vi "VI Tree.vi"   [LabVIEW 2010, in "Fluke 884X Series.lvlib"]
doc: "This is the instrument driver for the Fluke 8845 and 8846 digital multimeter."
uses:
  <instrlib>/Fluke 884X Series/Fluke 884X Series.lvlib
  <instrlib>/Fluke 884X Series/Public/Data/Read (Multiple Points).vi
panel:
  # "(c) 2007 National Instruments.  ALL RIGHTS RESERVED."
  # "SEE DIAGRAM\nFOR VI Tree"
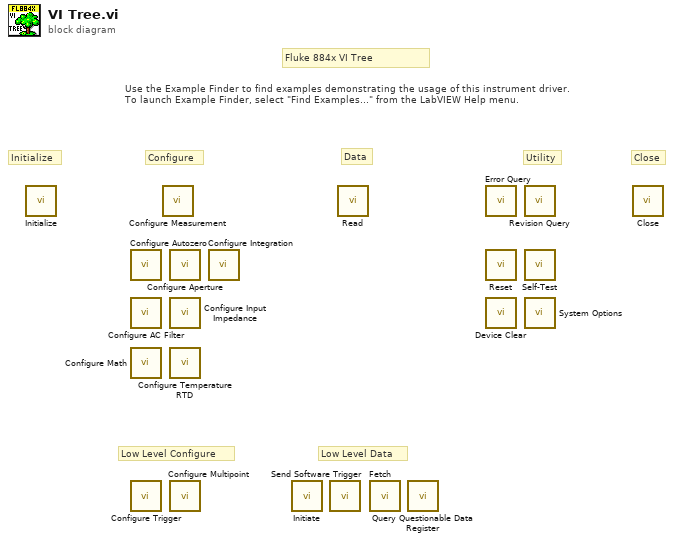
[diagram p0: block diagram]
diagram:
  # "Use the Example Finder to find examples demonstrating the usage of this instrument driver.\nTo launch Example Finder, select \"Find Examples...\" from the LabVIEW Help menu."
  # "Fluke 884x VI Tree"
  # "Low Level Configure"
  # "Low Level Data"
  # "Configure"
  # "Utility"
  # "Data"
  # "Close"
  # "Initialize"
  n1 = call <instrlib>:"Initialize.vi"() -> ()  [unwired: 10 in, 2 out]
  n2 = call <instrlib>:"Configure Autozero.vi"() -> ()  [unwired: 10 in, 2 out]
  n3 = call <instrlib>:"Configure AC Filter.vi"() -> ()  [unwired: 10 in, 2 out]
  n4 = call <instrlib>:"Configure Math.vi"() -> ()  [unwired: 14 in, 2 out]
  n5 = call <instrlib>:"Configure Trigger.vi"() -> ()  [unwired: 10 in, 2 out]
  n6 = call <instrlib>:"Configure Measurement.vi"() -> ()  [unwired: 10 in, 2 out]
  n7 = call <instrlib>:"Configure Aperture.vi"() -> ()  [unwired: 10 in, 2 out]
  n8 = call <instrlib>:"Configure Input Impedance.vi"() -> ()  [unwired: 10 in, 2 out]
  n9 = call <instrlib>:"Configure Temperature RTD.vi"() -> ()  [unwired: 14 in, 2 out]
  n10 = call <instrlib>:"Configure Multipoint.vi"() -> ()  [unwired: 10 in, 2 out]
  n11 = call <instrlib>:"Configure Integration.vi"() -> ()  [unwired: 10 in, 2 out]
  n12 = call <instrlib>:"Initiate.vi"() -> ()  [unwired: 10 in, 2 out]
  n13 = call <instrlib>:"Send Software Trigger.vi"() -> ()  [unwired: 10 in, 2 out]
  n14 = call-poly <instrlib>:"Read.vi"() -> ()  [unwired: 9 in, 3 out]
  n15 = call <instrlib>:"Fetch.vi"() -> ()  [unwired: 9 in, 3 out]
  n16 = call <instrlib>:"Query Questionable Data Register.vi"() -> ()  [unwired: 9 in, 3 out]
  n17 = call <instrlib>:"Error Query.vi"() -> ()  [unwired: 8 in, 4 out]
  n18 = call <instrlib>:"Reset.vi"() -> ()  [unwired: 10 in, 2 out]
  n19 = call <instrlib>:"Device Clear.vi"() -> ()  [unwired: 10 in, 2 out]
  n20 = call <instrlib>:"Revision Query.vi"() -> ()  [unwired: 8 in, 4 out]
  n21 = call <instrlib>:"Self-Test.vi"() -> ()  [unwired: 8 in, 4 out]
  n22 = call <instrlib>:"System Options.vi"() -> ()  [unwired: 10 in, 2 out]
  n23 = call <instrlib>:"Close.vi"() -> ()  [unwired: 11 in, 1 out]
